vi "Pack Bytes x8 (SubVI).vi"(0 "Input Valid?":bool, 2 "Data In":u8[](array[numeric])=[0, 0, 0, 0, 0, 0, 0, 0], 4 "Pixel Sync In":bool, 5 "N Bytes":u8) -> (14 "Output Valid?":bool, 17 "Pixel Sync Out":bool, 19 "Data Out":u64)   [LabVIEW 2015]
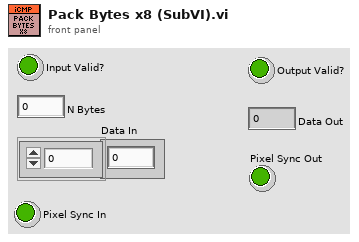
[diagram p1: front panel]
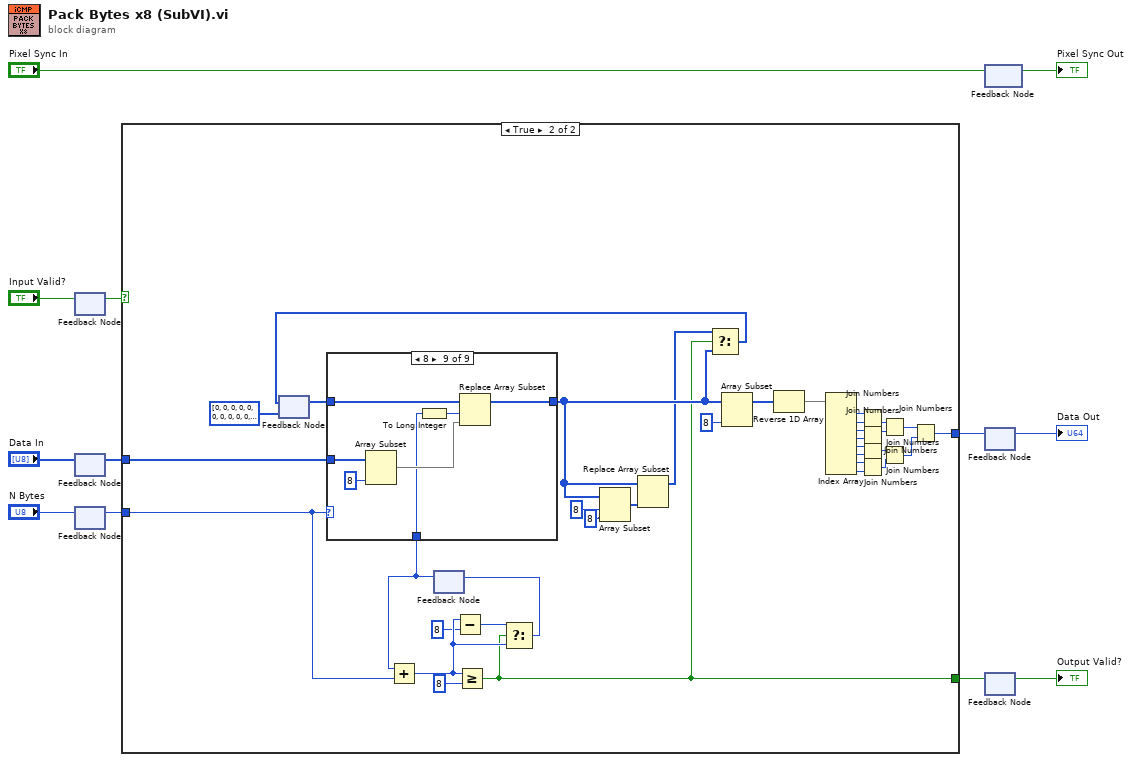
[diagram p0: block diagram]
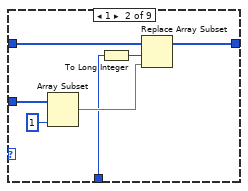
[diagram p4: hidden frame]
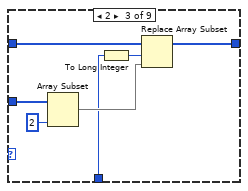
[diagram p5: hidden frame]
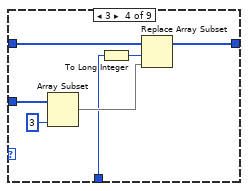
[diagram p6: hidden frame]
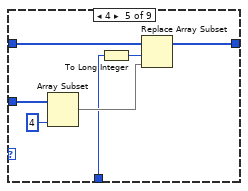
[diagram p7: hidden frame]
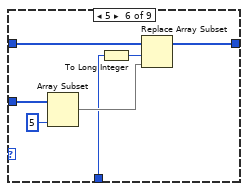
[diagram p8: hidden frame]
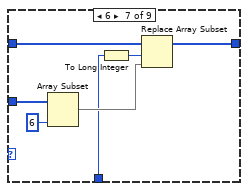
[diagram p9: hidden frame]
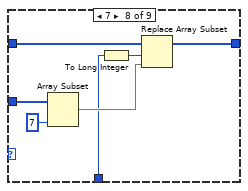
[diagram p10: hidden frame]
diagram:
  n1 = feedback-in #1("Input Valid?") -> ()
  n2 = feedback #1() -> (w11:bool)  [unwired: 1 in]
  n3 = feedback-in #2("Data In") -> ()
  n4 = feedback #2() -> (w8:u8[])  [unwired: 1 in]
  n5 = feedback-in #3("N Bytes") -> ()
  n6 = feedback #3() -> (w7:u8)  [unwired: 1 in]
  n7 = case shown="True" w11 {
    tunnel: w7 -> [_ w44]
    tunnel: w8 -> [_ w46]
    tunnel: [_ w18] -> w6
    tunnel: [_ w23] -> w5
    frame False {
    }
    frame True {
      n8 = feedback #4(u8[] [0, 0, 0, 0, 0, 0, 0, 0, 0, 0, 0, 0, 0, 0, 0, 0]) -> (w45:u8[])
      n9 = feedback #5() -> (w43:u8)  [unwired: 1 in]
      n10 = case shown="8" w44 {
        tunnel: w46 -> [_ w55 w62 w69 w76 w83 w90 w97 w104]
        tunnel: w45 -> [w48 w53 w60 w67 w74 w81 w88 w95 w102]
        tunnel: [w48 w51 w58 w65 w72 w79 w86 w93 w100] -> w19
        tunnel: w43 -> [_ w50 w57 w64 w71 w78 w85 w92 w99]
        frame 0, Default {
        }
        frame 1 {
          n11 = Array Subset(array=w55, length=1) -> (w54:u8[])  [unwired: 1 in]
          n12 = To Long Integer(number=w50) -> (32bit integer=w52:i32)
          n13 = Replace Array Subset(array=w53, new element=w54, index=w52) -> (w51:u8[])
        }
        frame 2 {
          n14 = Array Subset(array=w62, length=2) -> (w61:u8[])  [unwired: 1 in]
          n15 = To Long Integer(number=w57) -> (32bit integer=w59:i32)
          n16 = Replace Array Subset(array=w60, new element=w61, index=w59) -> (w58:u8[])
        }
        frame 3 {
          n17 = Array Subset(array=w69, length=3) -> (w68:u8[])  [unwired: 1 in]
          n18 = To Long Integer(number=w64) -> (32bit integer=w66:i32)
          n19 = Replace Array Subset(array=w67, new element=w68, index=w66) -> (w65:u8[])
        }
        frame 4 {
          n20 = Array Subset(array=w76, length=4) -> (w75:u8[])  [unwired: 1 in]
          n21 = To Long Integer(number=w71) -> (32bit integer=w73:i32)
          n22 = Replace Array Subset(array=w74, new element=w75, index=w73) -> (w72:u8[])
        }
        frame 5 {
          n23 = Array Subset(array=w83, length=5) -> (w82:u8[])  [unwired: 1 in]
          n24 = To Long Integer(number=w78) -> (32bit integer=w80:i32)
          n25 = Replace Array Subset(array=w81, new element=w82, index=w80) -> (w79:u8[])
        }
        frame 6 {
          n26 = Array Subset(array=w90, length=6) -> (w89:u8[])  [unwired: 1 in]
          n27 = To Long Integer(number=w85) -> (32bit integer=w87:i32)
          n28 = Replace Array Subset(array=w88, new element=w89, index=w87) -> (w86:u8[])
        }
        frame 7 {
          n29 = Array Subset(array=w97, length=7) -> (w96:u8[])  [unwired: 1 in]
          n30 = To Long Integer(number=w92) -> (32bit integer=w94:i32)
          n31 = Replace Array Subset(array=w95, new element=w96, index=w94) -> (w93:u8[])
        }
        frame 8 {
          n32 = Array Subset(array=w104, length=8) -> (w103:u8[])  [unwired: 1 in]
          n33 = To Long Integer(number=w99) -> (32bit integer=w101:i32)
          n34 = Replace Array Subset(array=w102, new element=w103, index=w101) -> (w100:u8[])
        }
      }
      n35 = Add(x=w43, y=w44) -> (x+y=w39:u8)
      n36 = Subtract(x=w39, y=u8 8) -> (x-y=w40:u8)
      n37 = Greater Or Equal?(x=w39, y=u8 8) -> (x >= y?=w18:bool)
      n38 = Select(t=w40, s=w18, f=w39) -> (s? t:f=w41:u8)
      n39 = feedback-in #5(w41) -> ()
      n40 = Array Subset(array=w19, index=8, length=8) -> (w20:u8[])
      n41 = Replace Array Subset(array=w19, new element=w20) -> (w17:u8[])  [unwired: 1 in]
      n42 = Select(t=w17, s=w18, f=w19) -> (s? t:f=w16:u8[])
      n43 = feedback-in #4(w16) -> ()
      n44 = Array Subset(array=w19, length=8) -> (w15:u8[])  [unwired: 1 in]
      n45 = Reverse 1D Array(array=w15) -> (reversed array=w13:u8[])
      n46 = Index Array(array=w13) -> (element #1=w36:u8, element #2=w37:u8, element #3=w34:u8, element #4=w35:u8, element #5=w33:u8, element #6=w32:u8, element #7=w31:u8, element #8=w30:u8)  [unwired: 8 in]
      n47 = Join Numbers(hi=w36, lo=w37) -> ((hi.lo)=w29:u16)
      n48 = Join Numbers(hi=w34, lo=w35) -> ((hi.lo)=w28:u16)
      n49 = Join Numbers(hi=w33, lo=w32) -> ((hi.lo)=w26:u16)
      n50 = Join Numbers(hi=w31, lo=w30) -> ((hi.lo)=w27:u16)
      n51 = Join Numbers(hi=w29, lo=w28) -> ((hi.lo)=w25:u32)
      n52 = Join Numbers(hi=w26, lo=w27) -> ((hi.lo)=w24:u32)
      n53 = Join Numbers(hi=w25, lo=w24) -> ((hi.lo)=w23:u64)
    }
  }
  n54 = feedback #6() -> (→"Pixel Sync Out":bool)  [unwired: 1 in]
  n55 = feedback-in #6("Pixel Sync In") -> ()
  n56 = feedback-in #7(w5) -> ()
  n57 = feedback #7() -> (→"Data Out":u64)  [unwired: 1 in]
  n58 = feedback-in #8(w6) -> ()
  n59 = feedback #8() -> (→"Output Valid?":bool)  [unwired: 1 in]
